vi "Create Registry.vi"(7 "type":refnum<class "NameRegistry.lvclass">, 8 "error in (no error)":errorcluster, 11 "Registry Configuration":T1) -> (0 "error out":errorcluster, 3 "Registry":refnum<data-value>)   [LabVIEW 2013, in "UniqueName.lvlib" / "NameRegistry.lvclass"]
uses:
  NameRegistry.lvclass
  Delimiter/Delimiter.lvclass
  RandomStringGenerator/RandomStringGenerator.lvclass
  UniquenessCriteria/UniquenessCriteria.lvclass
  StringIncrement/StringIncrement.lvclass
  RegistryConfiguration.ctl
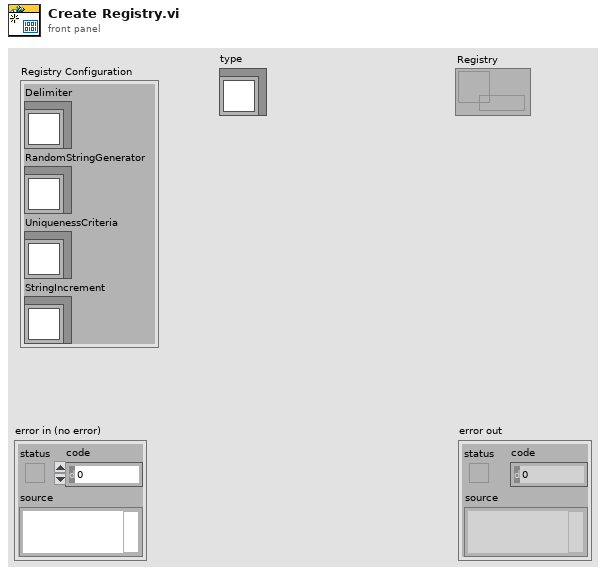
[diagram p1: front panel]
types:
  T1 = typedef "UniqueName.lvlib/NameRegistry.lvclass/RegistryConfiguration.ctl" = cluster{"Delimiter":refnum<class "Delimiter.lvclass">, "RandomStringGenerator":refnum<class "RandomStringGenerator.lvclass">, "UniquenessCriteria":refnum<class "UniquenessCriteria.lvclass">, "StringIncrement":refnum<class "StringIncrement.lvclass">}
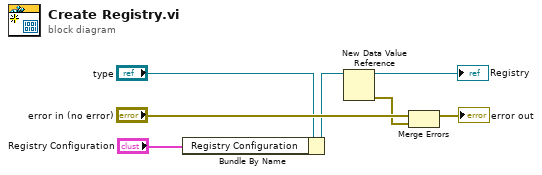
[diagram p0: block diagram]
diagram:
  n1 = Bundle By Name(cluster="type", "Registry Configuration"="Registry Configuration") -> (w3:refnum<class "NameRegistry.lvclass">)
  n2 = New Data Value Reference(data value=w3) -> (data value reference=→"Registry":refnum<data-value>, error out=w2:errorcluster)  [unwired: 1 in]
  n3 = Merge Errors("error in (no error)", w2) -> (→"error out":errorcluster)
